vi "Gain.vi"(11 "数组":dbl[](array[numeric])) -> (3 "K0":dbl)   [LabVIEW 2019]
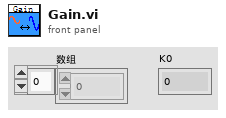
[diagram p1: front panel]
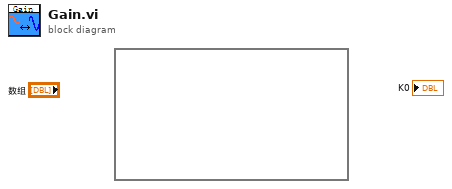
[diagram p0: block diagram]
diagram:
  n1 = formula code=""() -> ()
